vi "PWMin wrapper.vi"(10 "Value":bool, 11 "Timeout in":T2=40000) -> (3 "PWM out":T1)   [LabVIEW 2013]
uses:
  Typedefs/Time Out.ctl
  Typedefs/PWM.ctl
  <vilib>/NI Veristand/FPGA/NI_VS FPGA Support.lvlib
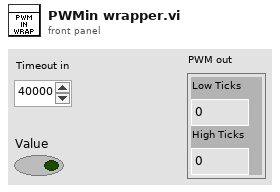
[diagram p1: front panel]
types:
  T1 = typedef "PWM.ctl" = cluster{"Low Ticks":u32, "High Ticks":u32}
  T2 = typedef "Time Out.ctl" = u32
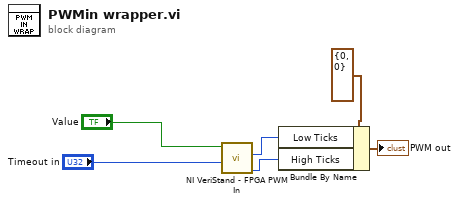
[diagram p0: block diagram]
diagram:
  n1 = call <vilib>:"NI VeriStand - FPGA PWM In.vi"("Time Out"="Timeout in", "Value"="Value") -> ("High time"=w4:u32, "Low Time"=w6:u32)  [unwired: 8 in]
  n2 = Bundle By Name(cluster=T1 {"Low Ticks"=0, "High Ticks"=0}, "Low Ticks"=w6, "High Ticks"=w4) -> (→"PWM out":T1)
